vi "Projectile.vi"() -> ()   [LabVIEW 2014]
uses:
  <vilib>/imath/engines/lvmath2/RunTimeEngine/Managers/WorkSpace/UID Generator.vi
  <vilib>/imath/engines/lvmath2/RunTimeEngine/RunTimeType/NIMS_RunTimeType_From StrictType (excl LVString).vi
  <instcachedir>/0/NIMS_RunTimeType_From StrictType (excl LVString)_15A5391EEA9C4AACB9955AC755B83D29.lvgen/NIMS_RunTimeType_From StrictType (excl LVString)_15A5391EEA9C4AACB9955AC755B83D29_000.vi
  <vilib>/imath/engines/lvmath2/RunTimeEngine/LocalVariableDefStatement/MC_LocalVariableDefStatement_Display.vi
  <vilib>/imath/engines/lvmath2/RunTimeEngine/Managers/SymbolTable/Clear UID.vi
  <vilib>/imath/engines/lvmath2/RunTimeEngine/NodeEndStatement/NIMS_NodeEndStatement_Output.vi
  <instcachedir>/0/NIMS_NodeEndStatement_Output_53EC0D466D134D7ABD903AC30B43404B.lvgen/NIMS_NodeEndStatement_Output_53EC0D466D134D7ABD903AC30B43404B_005.vi
  <vilib>/imath/engines/lvmath2/RunTimeEngine/ErrorHandling/NIMS_Finalize Error.vi
  <vilib>/imath/engines/lvmath2/RunTimeEngine/Managers/SymbolTable/NIMS_WorkSpace.lvlib
panel:
  out "XY Graph":cluster{"theta":dbl[], "R":dbl[]}(graph)
  in  "Launch Height (m)":dbl
  in  "Launch Speed (m/s)":dbl
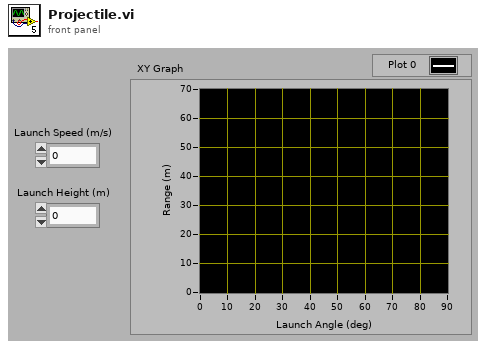
[diagram p1: front panel]
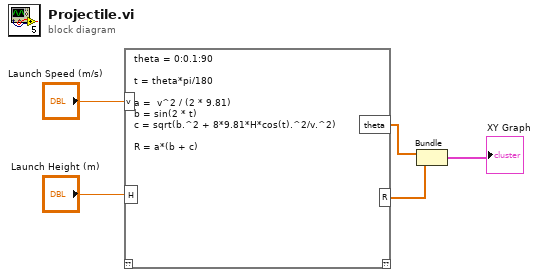
[diagram p0: block diagram]
diagram:
  n1 = mathscript code="theta = 0:0.1:90\n\nt = theta*pi/180\n\na =  v^2 / (2 * 9.81)\nb = sin(2 * t) \nc = sqrt(b.^2 + 8*9.81*H*cos(t).^2/v.^2)\n\nR = a*(b + c)"("v"="Launch Speed (m/s)", "H"="Launch Height (m)") -> ("R"=w5:dbl[], "theta"=w1:dbl[])  [unwired: 1 in, 1 out]
  n2 = Bundle("theta"=w1, "R"=w5) -> (→"XY Graph":cluster{"theta":dbl[], "R":dbl[]})  [unwired: 1 in]
